vi "FP_QTMTelegram_Read.vi"(8 "error in (no error)":errorcluster, 10 "timeout ms (25000)":i32=6000, 11 "connection ID in":refnum<k5>) -> (0 "error out":errorcluster, 1 "Data":string, 2 "Response type":i32, 3 "connection ID out":refnum<k5>, 4 "Response length":i32, 6 "error out 2":errorcluster)   [LabVIEW 2014]
panel:
  out "length 2":i32
  out "length":i32
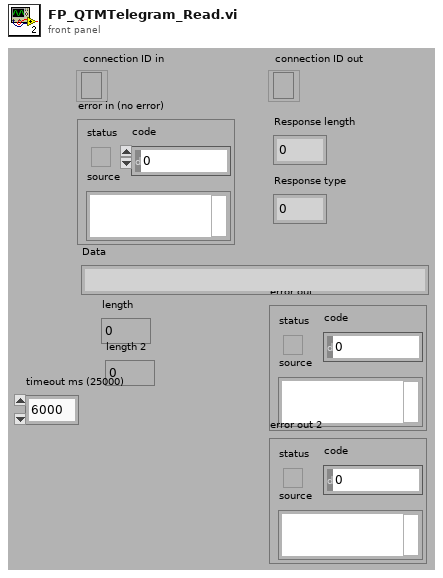
[diagram p1: front panel]
types:
  T1 = enum16{"Standard", "Buffered", "CRLF", "Immediate"}
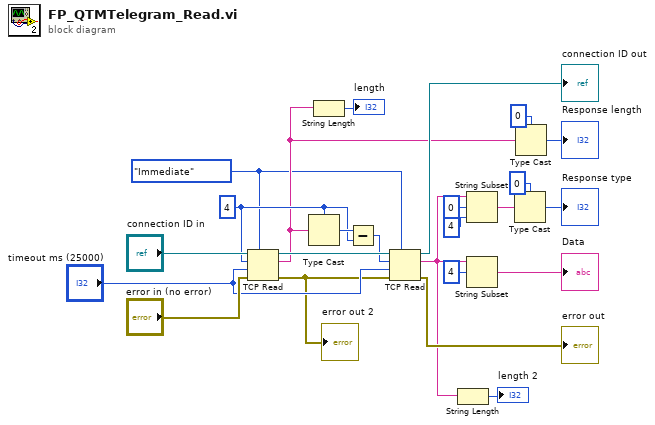
[diagram p0: block diagram]
diagram:
  w1 = T1."Immediate" ("mode (standard)")
  w18 = 4 ("bytes to read")
  n1 = TCP Read(connection ID="connection ID in", bytes to read=w18, error in (no error)="error in (no error)", 7:w1, 9:"timeout ms (25000)") -> (connection ID out=w20:refnum<k5>, data out=w6:string, error out=w2:errorcluster)
  "error out 2" <- w2
  n2 = Type Cast(type=w18, x=w6) -> (*(type *) &x=w19:i32)
  n3 = String Length(string=w6) -> (length=→"length":i32)
  n4 = Subtract(x=w19, y=w18) -> (x-y=w17:i32)
  n5 = TCP Read(connection ID=w20, bytes to read=w17, error in (no error)=w2, 7:w1, 9:"timeout ms (25000)") -> (connection ID out=→"connection ID out":refnum<k5>, data out=w4:string, error out=→"error out":errorcluster)
  n6 = String Length(string=w4) -> (length=→"length 2":i32)
  n7 = String Subset(string=w4, offset (0)=0, length (rest)=4 ("length (rest)")) -> (substring=w14:string)
  n8 = String Subset(string=w4, offset (0)=4) -> (substring=→"Data":string)  [unwired: 1 out]
  n9 = Type Cast(type=0 ("bytes to read"), x=w14) -> (*(type *) &x=→"Response type":i32)
  n10 = Type Cast(type=0 ("bytes to read"), x=w6) -> (*(type *) &x=→"Response length":i32)
